vi "Esophageal_FootPedal_InitializeTask.vi"(8 "error in (no error)":errorcluster) -> (0 "error out":errorcluster, 3 "Task Command":string)   [LabVIEW 2021]
uses:
  <resource>/objmgr/daqmx.rc
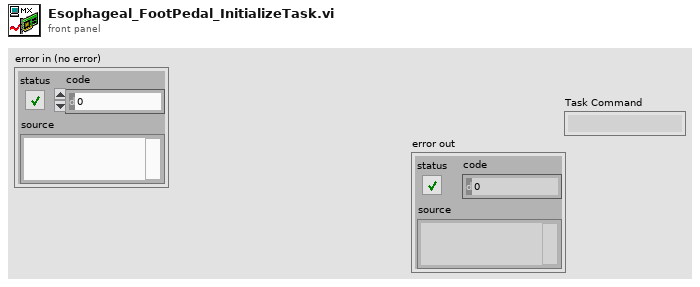
[diagram p1: front panel]
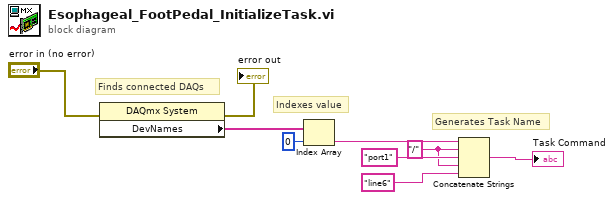
[diagram p0: block diagram]
diagram:
  w5 = "/" ("string")
  # "Generates Task Name"
  # "Indexes value"
  # "Finds connected DAQs"
  n1 = property class="DAQmx System"(error in="error in (no error)") -> (error out=→"error out":errorcluster, "DevNames"=w8:tag[])  [unwired: 1 in, 1 out]
  n2 = Index Array(array=w8, index=0) -> (element=w7:tag)
  n3 = Concatenate Strings(w7, w5, "port1" ("string"), w5, "line6" ("string")) -> (→"Task Command":string)
